vi "Submit.vi"(0 "VIP":refnum<class "VIP.lvclass">) -> (4 "VIP Out":refnum<class "VIP.lvclass">)   [LabVIEW 2017, in "CL_G3_VIComponentBuilder.lvlib" / "VIP.lvclass"]
doc: "Executes the commit behavior and moves the exported build spec to the build spec's original location, effectifely updating the build spec with the new build version information."
uses:
  VIP.lvclass
  C:/builds/Component BuilderBT/SrcDist/Exports/Exports/Export.lvclass
  Exports/Export.lvclass/Export.ctl
  Exports/Accessors/Read Commit behavior.vi
  Exports/Accessors/Read Exported Build Specification Path.vi
  Exports/Accessors/Read Export Build Specification.vi
  Exports/Accessors/Write Export Operation Errors.vi
  Commit Behavior/Commit/Commit.lvclass
  Exports/Export.lvclass
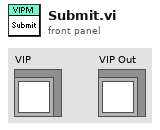
[diagram p1: front panel]
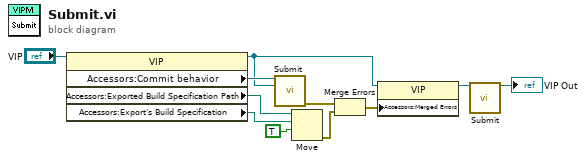
[diagram p0: block diagram]
diagram:
  n1 = property class="VIP"(reference="VIP") -> (reference out=w3:refnum<class "VIP.lvclass">, "Accessors:Commit behavior"=w4:refnum<class "Commit.lvclass">, "Accessors:Exported Build Specification Path"=w9:path, "Accessors:Export's Build Specification"=w8:path)  [unwired: 1 in, 1 out]
  n2 = call-dynamic "Submit.vi"("Commit in"=w4, "Export"=w3) -> ("error out"=w6:errorcluster)  [unwired: 12 in, 1 out]
  n3 = Move(source path=w9, 9:TRUE ("overwrite (F)"), 10:w8) -> (error out=w7:errorcluster)  [unwired: 2 in, 2 out]
  n4 = Merge Errors(w6, w7) -> (w1:errorcluster)
  n5 = property class="VIP"(reference=w3, "Accessors:Merged Errors"=w1) -> (reference out=w2:refnum<class "VIP.lvclass">)  [unwired: 1 in, 1 out]
  n6 = call-parent "Submit.vi"("Export In"=w2) -> ("Export Out"=→"VIP Out":refnum<class "VIP.lvclass">)  [unwired: 14 in]
